vi "f_9_Tf.vi"(0 "file path (IN)":path, 1 "Project #":string, 2 "Request #":string, 3 "TEST #":string, 5 "error in (no error)":errorcluster, 6 "ICE":dbl) -> (14 "file path (OUT)":path, 15 "Tf (ns)":dbl, 16 "DONE Tf":bool, 19 "error out":errorcluster)   [LabVIEW 2020]
uses:
  GlobIndSw1.vi
  <vilib>/Waveform/WDTOps.llb/WDT Waveform Duration DBL.vi
  <vilib>/Waveform/WDTOps.llb/WDT Get Waveform Subset DBL.vi
  <vilib>/measure/mamon.llb/Trigger Detection for 1 Channel.vi
  <vilib>/Analysis/NI_AALBase.lvlib
  <vilib>/measure/NI_MAPro.lvlib
panel:
  in  "Decision ?":bool
  out "10% Ice":dbl
  out "90% Ice":dbl
  out "Cursor b : Channel 1":dbl
  out "Cursor a : Channel 1":dbl
  out "Waveform Graph":waveform(dbl)[](graph)
  out "OFF Region":waveform(dbl)[](graph) caption="Tf (ns)"
  # "Tf: from 90% Ice to 10% Ice"
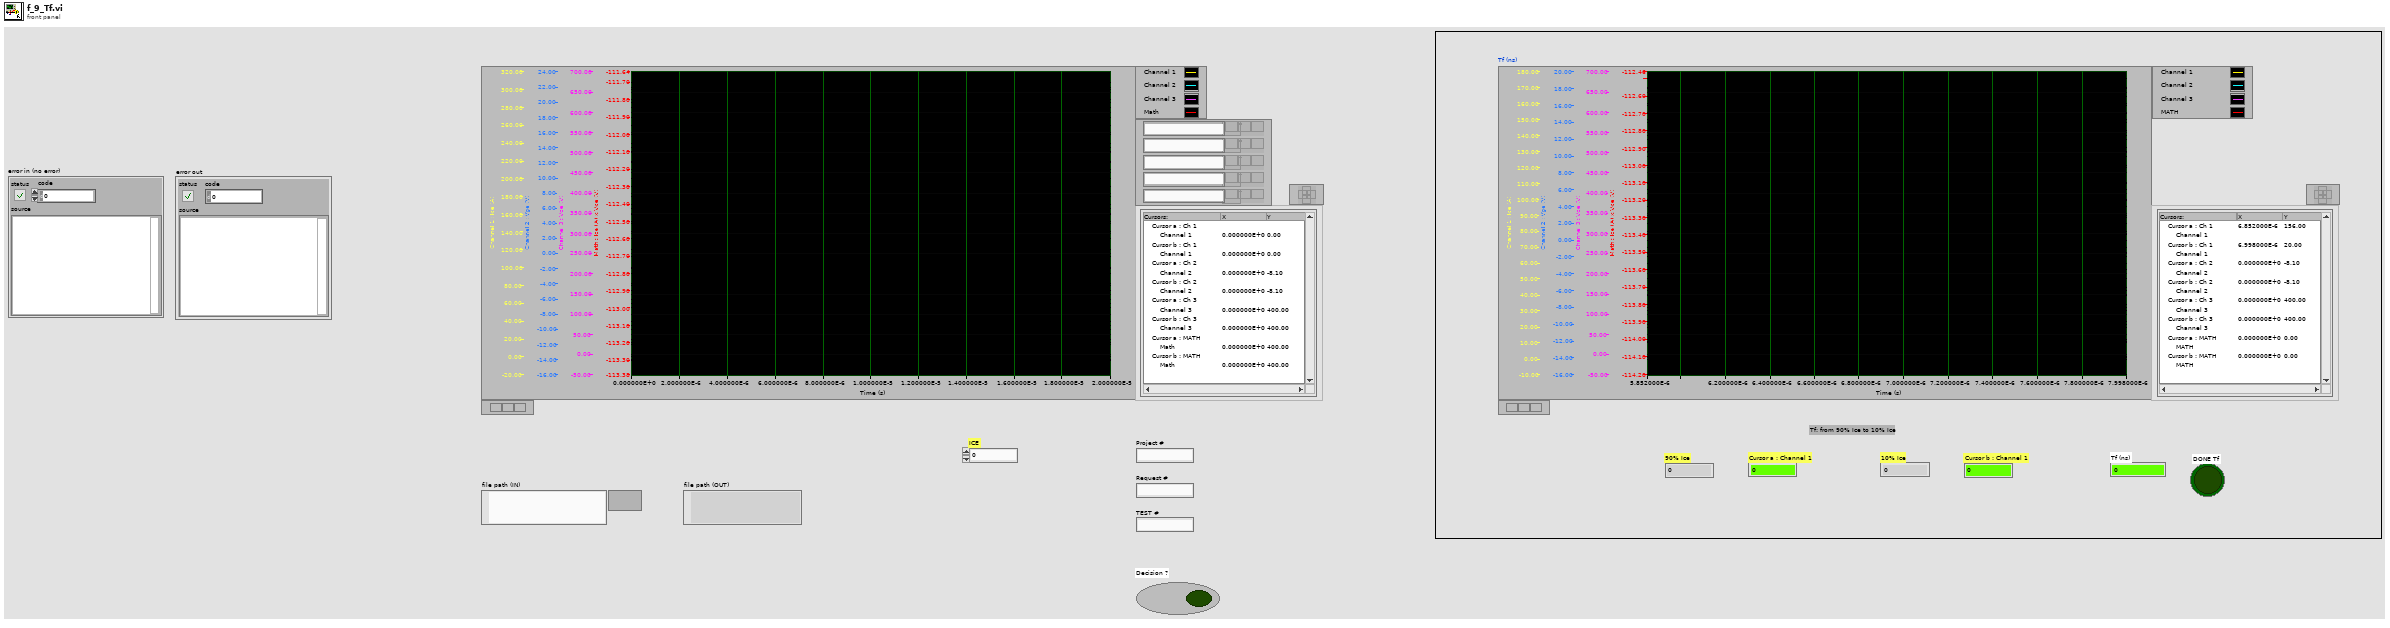
[diagram p1: front panel]
types:
  T1 = enum32{"Invalid", "Standard", "Closed", "Hidden", "Minimized", "Maximized"}
  T2 = typedef "imagedata.ctl" = cluster{"image type":i32, "image depth":i32, "image":u8[], "mask":u8[], "colors":u32[], "Rectangle":cluster{"left":i16, "top":i16, "right":i16, "bottom":i16}}
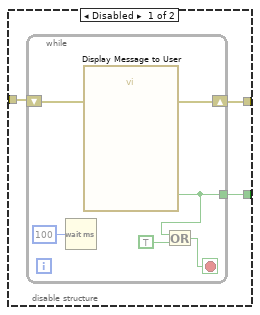
[diagram p2: hidden frame]
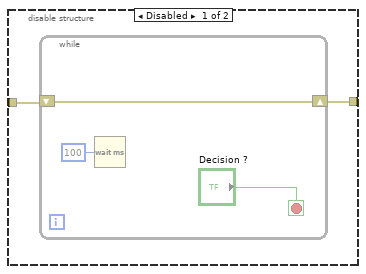
[diagram p7: hidden frame]
diagram:
  w1 = 0.0 ("Cursor a : Channel 1")
  w3 = errorcluster {"status"=FALSE, "code"=0, "source"=""} ("error out")
  w2 = FALSE ("DONE Tdon")
  w4 = waveform(dbl)[] [] ("Waveform Graph")
  n1 = local write "error out"(w3) -> ()
  n2 = local write "error in (no error)"(w3) -> ()
  n3 = local write "Cursor a : Channel 1"(w1) -> ()
  n4 = local write "Cursor b : Channel 1"(w1) -> ()
  n5 = local write "DONE Tf"(w2) -> ()
  n6 = local write "Waveform Graph"(w4) -> ()
  n7 = local write "OFF Region"(w4) -> ()
  n8 = local write "Decision ?"(w2) -> ()
  n9 = local write "Tf (ns)"(w1) -> ()
  n10 = flat-sequence {
    tunnel: ["file path (IN)"] -> w10
    tunnel: [w11] -> w9
    tunnel: [w22] -> w8
    tunnel: [w21] -> w7
    tunnel: w10 -> [w20]
    tunnel: w9 -> [w19]
    tunnel: w8 -> [w267]
    tunnel: [w266] -> w6
    tunnel: w7 -> [w266]
    tunnel: [w265] -> w5
    tunnel: w6 -> [w281]
    tunnel: w5 -> [w280]
    frame #0 {
      n11 = control-ref of="This VI"() -> (w17:refnum<vi>)
      n12 = invoke class="VI" method="FP.Open"(reference=w17, error in="error in (no error)", "Activate"=TRUE ("Activate?"), "State"=T1."Maximized") -> (error out=w18:errorcluster)  [unwired: 1 in, 4 out]
      n13 = property class="VI"(reference=w17, error in=w18, "Front Panel.Closeable"=TRUE ("Front Panel Window:Closeable")) -> (error out=w11:errorcluster)  [unwired: 1 out]
    }
    frame #1 {
      n14 = while {
        shift-right: [w28] -> w22
        shift-left: w19 -> [w27]
        tunnel: [w24] -> w21
        tunnel: w20 -> [w23]
        stop <- w29 stop-if-true
        n15 = flat-sequence {
          tunnel: w27 -> [w61]
          tunnel: [w61] -> w26
          tunnel: [w56] -> w25
          tunnel: w23 -> [w56]
          tunnel: [w63] -> w44
          tunnel: [w82] -> w43
          tunnel: [w72] -> w42
          tunnel: w26 -> [w158]
          tunnel: w25 -> [w152]
          tunnel: w44 -> [w196]
          tunnel: w43 -> [w206]
          tunnel: [w213] -> w41
          tunnel: w42 -> [w222]
          tunnel: [w222] -> w40
          tunnel: [w197] -> w39
          tunnel: [w204] -> w38
          tunnel: w41 -> [w241]
          tunnel: [w240] -> w37
          tunnel: w40 -> [w242]
          tunnel: [w242] -> w36
          tunnel: w39 -> [w234]
          tunnel: [w234] -> w35
          tunnel: w38 -> [w235]
          tunnel: [w235] -> w34
          tunnel: w37 -> [w244]
          tunnel: w36 -> [w250]
          tunnel: [w250] -> w33
          tunnel: w35 -> [w248]
          tunnel: w34 -> [w247]
          tunnel: [w244] -> w32
          tunnel: w33 -> [w255]
          tunnel: w32 -> [w257]
          tunnel: [w256] -> w31
          tunnel: [w255] -> w24
          frame #0 {
            w59 = 0.0 ("Cursor a : Channel 1")
            w58 = FALSE ("DONE Tdon")
            w57 = waveform(dbl)[] [] ("Waveform Graph")
            n16 = local write "Cursor a : Channel 1"(w59) -> ()
            n17 = local write "Cursor b : Channel 1"(w59) -> ()
            n18 = local write "DONE Tf"(w58) -> ()
            n19 = Wait (ms)(milliseconds to wait=u32 400) -> ()  [unwired: 1 out]
            n20 = local write "Waveform Graph"(w57) -> ()
            n21 = local write "OFF Region"(w57) -> ()
            n22 = local write "Decision ?"(w58) -> ()
            n23 = local write "Tf (ns)"(w59) -> ()
          }
          frame #1 {
            w66 = 0.0 ("start samples/time")
            w133 = u16 1 items=["Samples", "Relative Time"] ("start/duration format")
            w144 = u16 1 items=["Samples", "Relative Time"] ("start/duration format")
            w145 = u16 1 items=["Samples", "Relative Time"] ("start/duration format")
            # "Channel 1"
            # "Channel 3"
            # "Channel 2"
            # "dt"
            # "Ch2"
            # "Ch1"
            n24 = call "3_ReadDatatoWaveform.vi"("error in (no error)"=w158, "file path (IN)"=w152) -> ("error out"=w68:errorcluster, "Waveform Graph"=→"Waveform Graph":waveform(dbl)[], "file path (OUT)"=w72:path, "dt"=w153:dbl, "Ch 2 Data"=w150:dbl[], "Ch 3 Data"=w154:dbl[], "Ch 1 Data"=w151:dbl[])  [unwired: 3 in]
            n25 = To Time Stamp(1:0.0 ("number")) -> (0:w155:timestamp)
            n26 = disable-structure shown="Enabled" {
              disable-tunnel: w155 -> [w186 _]
              disable-tunnel: w153 -> [w185 _]
              disable-tunnel: w154 -> [w184 _]
              disable-tunnel: [w183 _] -> w131
              frame Enabled {
                # "Channel 3"
                n27 = Bundle By Name("Y"=w184, "dt"=w185, "t0"=w186) -> (w183:waveform(dbl))  [unwired: 1 in]
              }
              frame Disabled {
              }
            }
            n28 = disable-structure shown="Enabled" {
              disable-tunnel: w155 -> [w178 _]
              disable-tunnel: w153 -> [w177 _]
              disable-tunnel: w151 -> [w176 _]
              disable-tunnel: [w175 _] -> w67
              frame Enabled {
                # "Channel 1"
                n29 = Bundle By Name("Y"=w176, "dt"=w177, "t0"=w178) -> (w175:waveform(dbl))  [unwired: 1 in]
              }
              frame Disabled {
              }
            }
            n30 = disable-structure shown="Enabled" {
              disable-tunnel: w155 -> [w182 _]
              disable-tunnel: w153 -> [w181 _]
              disable-tunnel: w150 -> [w180 _]
              disable-tunnel: [w179 _] -> w132
              frame Enabled {
                # "Channel 2"
                n31 = Bundle By Name("Y"=w180, "dt"=w181, "t0"=w182) -> (w179:waveform(dbl))  [unwired: 1 in]
              }
              frame Disabled {
              }
            }
            n32 = Wait (ms)(milliseconds to wait=u32 400) -> ()  [unwired: 1 out]
            n33 = call <vilib>:"Beep.vi"("use system alert? (T)"=FALSE, "duration (msec)"=u32 200, "frequency (Hz)"=u32 2000) -> ()  [unwired: 9 in]
            n34 = disable-structure shown="Enabled" {
              disable-tunnel: w67 -> [w171 _]
              disable-tunnel: w68 -> [w163 _]
              disable-tunnel: [w162 _] -> w65
              disable-tunnel: [w161 _] -> w63
              disable-tunnel: w66 -> [w160 _]
              frame Enabled {
                w165 = u16 1 items=["Samples", "Relative Time"] ("start/duration format")
                # "Channel 1 - Filtered"
                # "Median"
                n35 = global read "GlobIndSw1.vi" "Median Filter Rank"() -> (w159:i32)
                n36 = Unbundle By Name(w171) -> ("Y"=w174:dbl[], "dt"=w172:dbl)
                n37 = call <vilib>:"Median Filter.vi"("right rank"=w159, "left rank"=w159, "X"=w174) -> ("Filtered X"=w173:dbl[])  [unwired: 7 in, 1 out]
                n38 = Bundle By Name("Y"=w173, "dt"=w172) -> (w164:waveform(dbl))  [unwired: 1 in]
                n39 = call-poly <vilib>:"Waveform Duration.vi"("error in (no error)"=w163, "waveform in"=w164) -> ("error out"=w168:errorcluster, "duration"=w170:dbl, "waveform out"=w169:waveform(dbl))  [unwired: 7 in]
                n40 = Divide(x=w170, y=2.0) -> (x/y=w167:dbl)
                n41 = call-poly <vilib>:"Get Waveform Subset.vi"("start/duration format"=w165, "error in (no error)"=w168, "duration"=w167, "start samples/time"=w160, "waveform in"=w169) -> ("error out"=w162:errorcluster, "waveform out"=w161:waveform(dbl))  [unwired: 1 in, 2 out]
              }
              frame Disabled {
              }
            }
            n42 = call-poly <vilib>:"Waveform Duration.vi"("error in (no error)"=w68, "waveform in"=w131) -> ("error out"=w138:errorcluster, "duration"=w135:dbl, "waveform out"=w137:waveform(dbl))  [unwired: 7 in]
            n43 = call-poly <vilib>:"Waveform Duration.vi"("error in (no error)"=w68, "waveform in"=w132) -> ("error out"=w139:errorcluster, "duration"=w142:dbl, "waveform out"=w140:waveform(dbl))  [unwired: 7 in]
            n44 = call-poly <vilib>:"Waveform Duration.vi"("error in (no error)"=w68, "waveform in"=w67) -> ("error out"=w149:errorcluster, "duration"=w146:dbl, "waveform out"=w148:waveform(dbl))  [unwired: 7 in]
            n45 = Divide(x=w135, y=2.0) -> (x/y=w134:dbl)
            n46 = Divide(x=w142, y=2.0) -> (x/y=w143:dbl)
            n47 = Divide(x=w146, y=2.0) -> (x/y=w128:dbl)
            n48 = call-poly <vilib>:"Get Waveform Subset.vi"("start/duration format"=w133, "error in (no error)"=w138, "duration"=w134, "start samples/time"=w66, "waveform in"=w137) -> ("error out"=w125:errorcluster, "waveform out"=w130:waveform(dbl))  [unwired: 1 in, 2 out]
            n49 = call-poly <vilib>:"Get Waveform Subset.vi"("start/duration format"=w144, "error in (no error)"=w139, "duration"=w143, "start samples/time"=w66, "waveform in"=w140) -> ("error out"=w126:errorcluster, "waveform out"=w84:waveform(dbl))  [unwired: 1 in, 2 out]
            n50 = call-poly <vilib>:"Get Waveform Subset.vi"("start/duration format"=w145, "error in (no error)"=w149, "duration"=w128, "start samples/time"=w66, "waveform in"=w148) -> ("error out"=w127:errorcluster, "waveform out"=w83:waveform(dbl))  [unwired: 1 in, 2 out]
            n51 = Build Array(w83, w84, w130, waveform(dbl) {"t0"=timestamp(0 s since 1904-01-01), "dt"=1.0, "Y"=[]} ("element")) -> (→"OFF Region":waveform(dbl)[])
            n52 = Merge Errors(w127, w126, w125, w65) -> (w80:errorcluster)
            n53 = property on="OFF Region" class="WFGraph (strict)"(error in=w80) -> (error out=w79:errorcluster, "Width"=w78:u32)  [unwired: 1 in, 1 out]
            n54 = property on="OFF Region" class="WFGraph (strict)"(error in=w79, "Caption.Justify"=enum16{"Left", "Center", "Right"}."Left" ("Caption.Justification"), "Caption.Width"=w78, "Caption.FontBold"=TRUE ("Caption.Font:Bold"), "Caption.FontColor"=u32 16860 ("Caption.Font:Color"), "Caption.FontSize"=u32 24 ("Caption.Font:Size"), "Caption.Text"="Tf (ns)") -> (error out=w74:errorcluster)  [unwired: 1 in, 1 out]
            n55 = property on="OFF Region" class="WFGraph (strict)"(error in=w74, "XScale.Offset"=w66) -> (error out=w108:errorcluster)  [unwired: 1 in, 1 out]
            n56 = property on="OFF Region" class="WFGraph (strict)"(error in=w108, "Active Cursor"=u32 0, "Cursor.Cursor X"=0.0 ("Cursor.Cursor Position:Cursor X"), "Cursor.Cursor Y"=0.0 ("Cursor.Cursor Position:Cursor Y"), "Cursor.Visible"=FALSE) -> (error out=w107:errorcluster)  [unwired: 1 in, 1 out]
            n57 = property on="OFF Region" class="WFGraph (strict)"(error in=w107, "Active Cursor"=u32 1, "Cursor.Cursor X"=0.0 ("Cursor.Cursor Position:Cursor X"), "Cursor.Cursor Y"=0.0 ("Cursor.Cursor Position:Cursor Y"), "Cursor.Visible"=FALSE) -> (error out=w106:errorcluster)  [unwired: 1 in, 1 out]
            n58 = property on="OFF Region" class="WFGraph (strict)"(error in=w106, "Active Cursor"=u32 2, "Cursor.Cursor X"=0.0 ("Cursor.Cursor Position:Cursor X"), "Cursor.Cursor Y"=0.0 ("Cursor.Cursor Position:Cursor Y"), "Cursor.Visible"=FALSE) -> (error out=w105:errorcluster)  [unwired: 1 in, 1 out]
            n59 = property on="OFF Region" class="WFGraph (strict)"(error in=w105, "Active Cursor"=u32 3, "Cursor.Cursor X"=0.0 ("Cursor.Cursor Position:Cursor X"), "Cursor.Cursor Y"=0.0 ("Cursor.Cursor Position:Cursor Y"), "Cursor.Visible"=FALSE) -> (error out=w88:errorcluster)  [unwired: 1 in, 1 out]
            n60 = property on="OFF Region" class="WFGraph (strict)"(error in=w88, "Active Cursor"=u32 4, "Cursor.Cursor X"=0.0 ("Cursor.Cursor Position:Cursor X"), "Cursor.Cursor Y"=0.0 ("Cursor.Cursor Position:Cursor Y"), "Cursor.Visible"=FALSE) -> (error out=w87:errorcluster)  [unwired: 1 in, 1 out]
            n61 = property on="OFF Region" class="WFGraph (strict)"(error in=w87, "Active Cursor"=u32 5, "Cursor.Cursor X"=0.0 ("Cursor.Cursor Position:Cursor X"), "Cursor.Cursor Y"=0.0 ("Cursor.Cursor Position:Cursor Y"), "Cursor.Visible"=FALSE) -> (error out=w86:errorcluster)  [unwired: 1 in, 1 out]
            n62 = property on="OFF Region" class="WFGraph (strict)"(error in=w86, "Active Cursor"=u32 6, "Cursor.Cursor X"=0.0 ("Cursor.Cursor Position:Cursor X"), "Cursor.Cursor Y"=0.0 ("Cursor.Cursor Position:Cursor Y"), "Cursor.Visible"=FALSE) -> (error out=w85:errorcluster)  [unwired: 1 in, 1 out]
            n63 = property on="OFF Region" class="WFGraph (strict)"(error in=w85, "Active Cursor"=u32 7, "Cursor.Cursor X"=0.0 ("Cursor.Cursor Position:Cursor X"), "Cursor.Cursor Y"=0.0 ("Cursor.Cursor Position:Cursor Y"), "Cursor.Visible"=FALSE) -> (error out=w82:errorcluster)  [unwired: 1 in, 1 out]
          }
          frame #2 {
            w200 = u16 0 items=["Falling Edge", "Rising Edge"] ("trigger slope")
            w201 = u16 1 items=["Index", "Time"] ("location mode")
            w208 = u16 0 items=["Falling Edge", "Rising Edge"] ("trigger slope")
            w209 = u16 1 items=["Index", "Time"] ("location mode")
            # "Cursor a : Channel 1"
            # "Cursor b : Channel 1"
            # "Cursor b : Channel 1"
            # "Cursor a : Channel 1"
            # "Cursor b : Channel 1"
            # "Cursor a : Channel 1"
            # "End Time 1st Cursor"
            # "End Time 2nd Cursor"
            # "1st PARAMETER : 90% Ice"
            # "Channel 1"
            # "2nd PARAMETER : 10% Ice"
            # "Channel 1"
            n64 = Wait (ms)(milliseconds to wait=u32 500) -> ()  [unwired: 1 out]
            n65 = call <vilib>:"Beep.vi"("use system alert? (T)"=FALSE, "duration (msec)"=u32 200, "frequency (Hz)"=u32 2000) -> ()  [unwired: 9 in]
            n66 = Divide(x=90.0, y=100.0) -> (x/y=w232:dbl)
            n67 = Multiply(x=w232, y="ICE") -> (x*y=w205:dbl)
            "90% Ice" <- w205
            n68 = Add(x=w205, y=0.2) -> (x+y=w192:dbl)
            n69 = Divide(x=w192, y=10.0) -> (x/y=w191:dbl)
            n70 = call-poly <vilib>:"Basic Level Trigger Detection.vi"("signal in"=w196, "level"=w192, "hysteresis"=w191, "location mode"=w209, "error in (no error)"=w206, "trigger slope"=w208) -> ("trigger location"=w204:dbl, "error out"=w203:errorcluster)  [unwired: 7 in, 1 out]
            n71 = property on="OFF Region" class="WFGraph (strict)"(error in=w203, "Active Cursor"=u32 0, "Cursor.Cursor X"=w204, "Cursor.Visible"=TRUE, "Cursor.Cursor Name Visible"=TRUE) -> (error out=w217:errorcluster)  [unwired: 1 in, 1 out]
            n72 = property on="OFF Region" class="WFGraph (strict)"(error in=w217, "Active Cursor"=u32 0) -> (error out=w195:errorcluster, "Cursor.Cursor Y"=→"Cursor a : Channel 1":dbl)  [unwired: 1 in, 1 out]
            n73 = Divide(x=10.0, y=100.0) -> (x/y=w229:dbl)
            n74 = Multiply(x=w229, y="ICE") -> (x*y=w194:dbl)
            "10% Ice" <- w194
            n75 = Add(x=w194, y=0.2) -> (x+y=w189:dbl)
            n76 = Divide(x=w189, y=10.0) -> (x/y=w188:dbl)
            n77 = call-poly <vilib>:"Basic Level Trigger Detection.vi"("signal in"=w196, "level"=w189, "hysteresis"=w188, "location mode"=w201, "error in (no error)"=w195, "trigger slope"=w200) -> ("trigger location"=w197:dbl, "error out"=w198:errorcluster)  [unwired: 7 in, 1 out]
            n78 = property on="OFF Region" class="WFGraph (strict)"(error in=w198, "Active Cursor"=u32 1, "Cursor.Cursor X"=w197, "Cursor.Visible"=TRUE, "Cursor.Cursor Name Visible"=TRUE) -> (error out=w214:errorcluster)  [unwired: 1 in, 1 out]
            n79 = property on="OFF Region" class="WFGraph (strict)"(error in=w214, "Active Cursor"=u32 1) -> (error out=w213:errorcluster, "Cursor.Cursor Y"=→"Cursor b : Channel 1":dbl)  [unwired: 1 in, 1 out]
          }
          frame #3 {
            # "2nd Cursor"
            # "1st Cursor"
            n80 = Subtract(x=w235, y=1e-06) -> (x-y=w236:dbl)
            n81 = Add(x=w234, y=1e-06) -> (x+y=w237:dbl)
            n82 = Wait (ms)(milliseconds to wait=u32 300) -> ()  [unwired: 1 out]
            n83 = property on="OFF Region" class="WFGraph (strict)"(error in=w241, "XScale.Minimum"=w236, "XScale.Maximum"=w237) -> (error out=w240:errorcluster)  [unwired: 1 in, 1 out]
          }
          frame #4 {
            # "ns"
            n84 = Subtract(x=w248, y=w247) -> (x-y=w246:dbl)
            n85 = Absolute Value(x=w246) -> (abs(x)=w245:dbl)
            n86 = Multiply(x=w245, y=1000000000.0) -> (x*y=→"Tf (ns)":dbl)
            n87 = Wait (ms)(milliseconds to wait=u32 300) -> ()  [unwired: 1 out]
            n88 = call <vilib>:"Beep.vi"("use system alert? (T)"=FALSE, "duration (msec)"=u32 200, "frequency (Hz)"=u32 2000) -> ()  [unwired: 9 in]
          }
          frame #5 {
            n89 = disable-structure shown="Enabled" {
              disable-tunnel: w257 -> [w259 w263]
              disable-tunnel: [w258 w263] -> w256
              frame Disabled {
                n90 = while {
                  shift-right: [w260] -> w258
                  shift-left: w259 -> [w260]
                  stop <- "Decision ?" stop-if-true
                  n91 = Wait (ms)(milliseconds to wait=u32 100) -> ()  [unwired: 1 out]
                }
              }
              frame Enabled {
              }
            }
          }
        }
        n92 = disable-structure shown="Enabled" {
          disable-tunnel: w31 -> [w47 w55]
          disable-tunnel: [w46 TRUE ("NO")] -> w29
          disable-tunnel: [w45 w55] -> w28
          frame Disabled {
            n93 = while {
              tunnel: [w49] -> w46
              shift-right: [w52] -> w45
              shift-left: w47 -> [w53]
              stop <- w51 stop-if-true
              n94 = Wait (ms)(milliseconds to wait=u32 100) -> ()  [unwired: 1 out]
              n95 = call "Display Message to User"("error in (no error)"=w53) -> ("error out"=w52:errorcluster, "NO"=w49:bool)  [unwired: 9 in]
              n96 = Or(x=w49, y=TRUE) -> (x .or. y?=w51:bool)
            }
          }
          frame Enabled {
          }
        }
        n97 = Wait (ms)(milliseconds to wait=u32 100) -> ()  [unwired: 1 out]
      }
    }
    frame #2 {
      w271 = "_"
      n98 = Wait (ms)(milliseconds to wait=u32 300) -> ()  [unwired: 1 out]
      n99 = invoke on="OFF Region" class="WFGraph (strict)" method="Get Image"(error in=w267) -> (error out=w273:errorcluster, "image data"=w276:T2)  [unwired: 5 in, 4 out]
      n100 = Concatenate Strings("C:\\Inductive_Switching_Project\\IndSw_Image\\" ("string"), "Project #", w271, "Request #", w271, "TEST #", w271, "Tf" ("string"), ".png" ("string")) -> (w277:string)
      n101 = String To Path(string=w277) -> (path=w275:path)
      n102 = call <vilib>:"Write PNG File.vi"("error in (no error)"=w273, "image data"=w276, "path to PNG file"=w275) -> ("error out"=w265:errorcluster)  [unwired: 7 in, 1 out]
      "DONE Tf" <- TRUE ("DONE Tdon")
    }
    frame #3 {
      n103 = disable-structure shown="Enabled" {
        disable-tunnel: w280 -> [w282 _]
        frame Enabled {
          n104 = control-ref of="This VI"() -> (w283:refnum<vi>)
          n105 = invoke class="VI" method="FP.Close"(reference=w283, error in=w282) -> ()  [unwired: 1 in, 3 out]
        }
        frame Disabled {
        }
      }
      "error out" <- w280
      "file path (OUT)" <- w281
    }
  }
